vi "Get Panel Indicator List.vi"(4 "error in":errorcluster, 7 "Call Level (3)":i32=3) -> (0 "error out":errorcluster {"code" format="%.0x"}, 2 "label list":string[](array[string]), 3 "indicator list":refnum<vi>[](array[refnum]))   [LabVIEW 2010]
doc: "This function gets a list of references to all control \"indicators\" on a calling VI front panel."
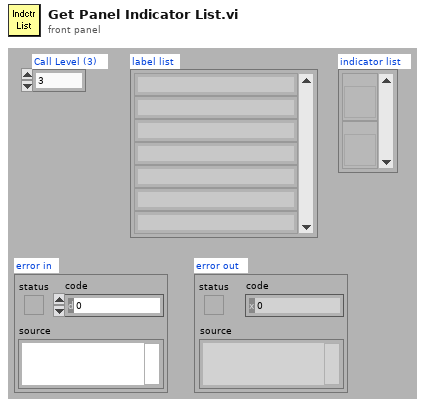
[diagram p1: front panel]
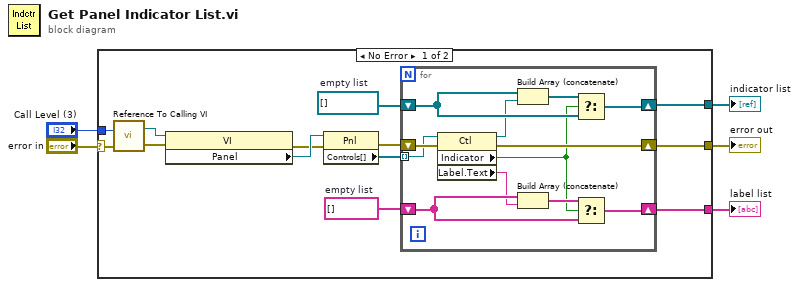
[diagram p0: block diagram]
diagram:
  n1 = case shown="No Error" "error in" {
    selector: "error in" -> [w10 w31]
    tunnel: [w12 w31] -> w5
    tunnel: "Call Level (3)" -> [w11 _]
    tunnel: [w9 _] -> w2
    tunnel: [w6 _] -> w1
    frame No Error {
      w7 = string[] []  # empty list
      w8 = refnum<vi>[] []  # empty list
      n2 = call "Reference To Calling VI.vi"("error in"=w10, "Call Level (2)"=w11) -> ("error out"=w15:errorcluster, "VI Reference"=w16:refnum<vi>)  [unwired: 1 in]
      n3 = property class="VI"(reference=w16, error in=w15) -> (error out=w17:errorcluster, "Panel"=w18:refnum<vi>)  [unwired: 1 out]
      n4 = property class="Pnl"(reference=w18, error in=w17) -> (error out=w13:errorcluster, "Controls[]"=w14:refnum<vi>[])  [unwired: 1 out]
      n5 = for {
        tunnel: w14 -> [w20] mode=indexing
        shift-right: [w29] -> w12
        shift-left: w13 -> [w30]
        shift-right: [w22] -> w6
        shift-left: w7 -> [w23]
        shift-right: [w26] -> w9
        shift-left: w8 -> [w25]
        n6 = property class="Ctl"(reference=w20, error in=w30) -> (reference out=w19:refnum<vi>, error out=w29:errorcluster, "Indicator"=w24:bool, "Label.Text"=w21:string)
        n7 = Build Array (concatenate)(w25, w19) -> (w27:refnum<vi>[])
        n8 = Build Array (concatenate)(w23, w21) -> (w28:string[])
        n9 = Select(t=w27, s=w24, f=w25) -> (s? t:f=w26:refnum<vi>[])
        n10 = Select(t=w28, s=w24, f=w23) -> (s? t:f=w22:string[])
      }
    }
    frame Error {
    }
  }
  "error out" <- w5
  "indicator list" <- w2
  "label list" <- w1
